vi "Instru.vi"(8 "错误输入（无错误）":errorcluster, 11 "VISA资源名称":refnum<visa-resource-name>="COM2") -> (0 "error out":errorcluster caption="错误输出")   [LabVIEW 2014]
uses:
  <vilib>/Instr/_visa.llb/VISA Configure Serial Port (Instr).vi
panel:
  out "温度":dbl
  out "电流通道":dbl
  out "电压通道":dbl
  out "实验类型":string
  out "示波器试验频率":dbl
  in  "实时数据停止":bool
  out "实时数据":dbl[](array[numeric])
  out "NegativeDutyCycle":dbl
  out "PositiveDutyCycle":dbl
  out "NegWidth":dbl
  out "PosWidth":dbl
  out "Falltime":dbl
  out "RiseTime":dbl
  out "ACRMS":dbl
  in  "x 2":bool
  out "FREQ":dbl
  out "MIN":dbl
  out "RMS":dbl
  out "AMP":dbl
  out "Max":dbl
  out "PK2PK":dbl
  out "PERIOD":dbl
  in  "一键查询":bool
  in  "停止 2":bool
  out "错误输出 2":errorcluster caption="错误输出"
  in  "停止":bool
  in  "自动采集":bool
  in  "查询":bool
  in  "选项卡控件":T1(tab)
  in  "保存数据与截图":bool
  out "二维图片":picture
  out "处理中":u8(slide) scale=0.0..100.0
  in  "选择通道":u16(ring) items=["电压通道", "电流通道"]
  out "表格控件":string[][](table)
  out "表格控件 2":string[][](table)
  out "表格控件 3":string[][](table)
  out "表格控件 11":string[][](table)
  out "表格控件 12":string[][](table)
  out "表格控件 13":string[][](table)
  out "表格控件 14":string[][](table)
  out "表格控件 15":string[][](table)
  out "表格控件 16":string[][](table)
  out "表格控件 17":string[][](table)
  in  "电流通道":enum32{"CH1", " 2"}(radio)
  in  "电压通道":T2(radio)
  in  "FTP":bool
  in  "复位":bool
  in  "查询仪表信息":bool
  out "仪表信息 2":string
  in  "地址":refnum<visa-resource-name>="DPO5054-C012667"
  # "示波器"
  # "查询各通道的参数值"
  # "结果显示"
  # "交流通道采集"
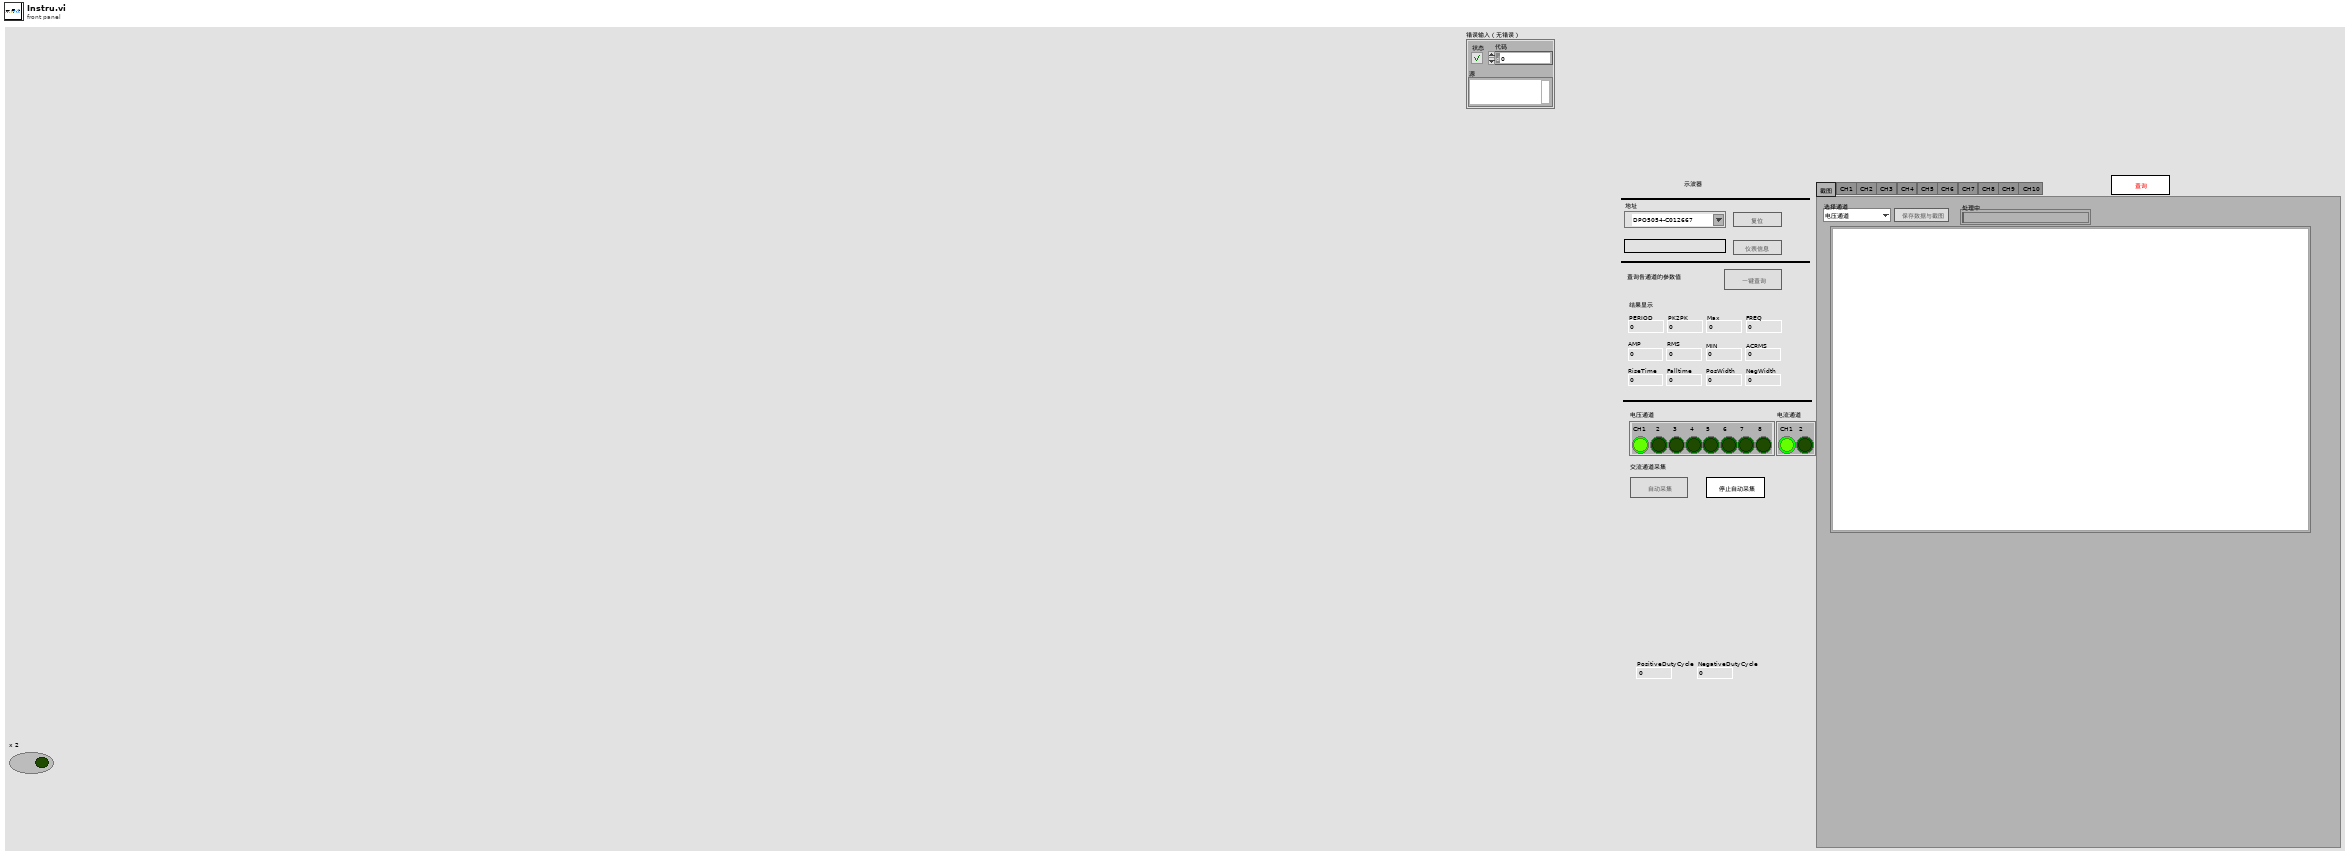
[diagram p1: front panel]
types:
  T1 = enum32{"截图", "CH1", "CH2", "CH3", "CH4", "CH5", "CH6", "CH7", "CH8", "CH9", "CH10"}
  T2 = enum32{"CH1", "2", "3", "4", " 5", " 6", " 7", " 8"}
  T3 = enum8{"Enabled", "Disabled", "Disabled and Grayed Out"}
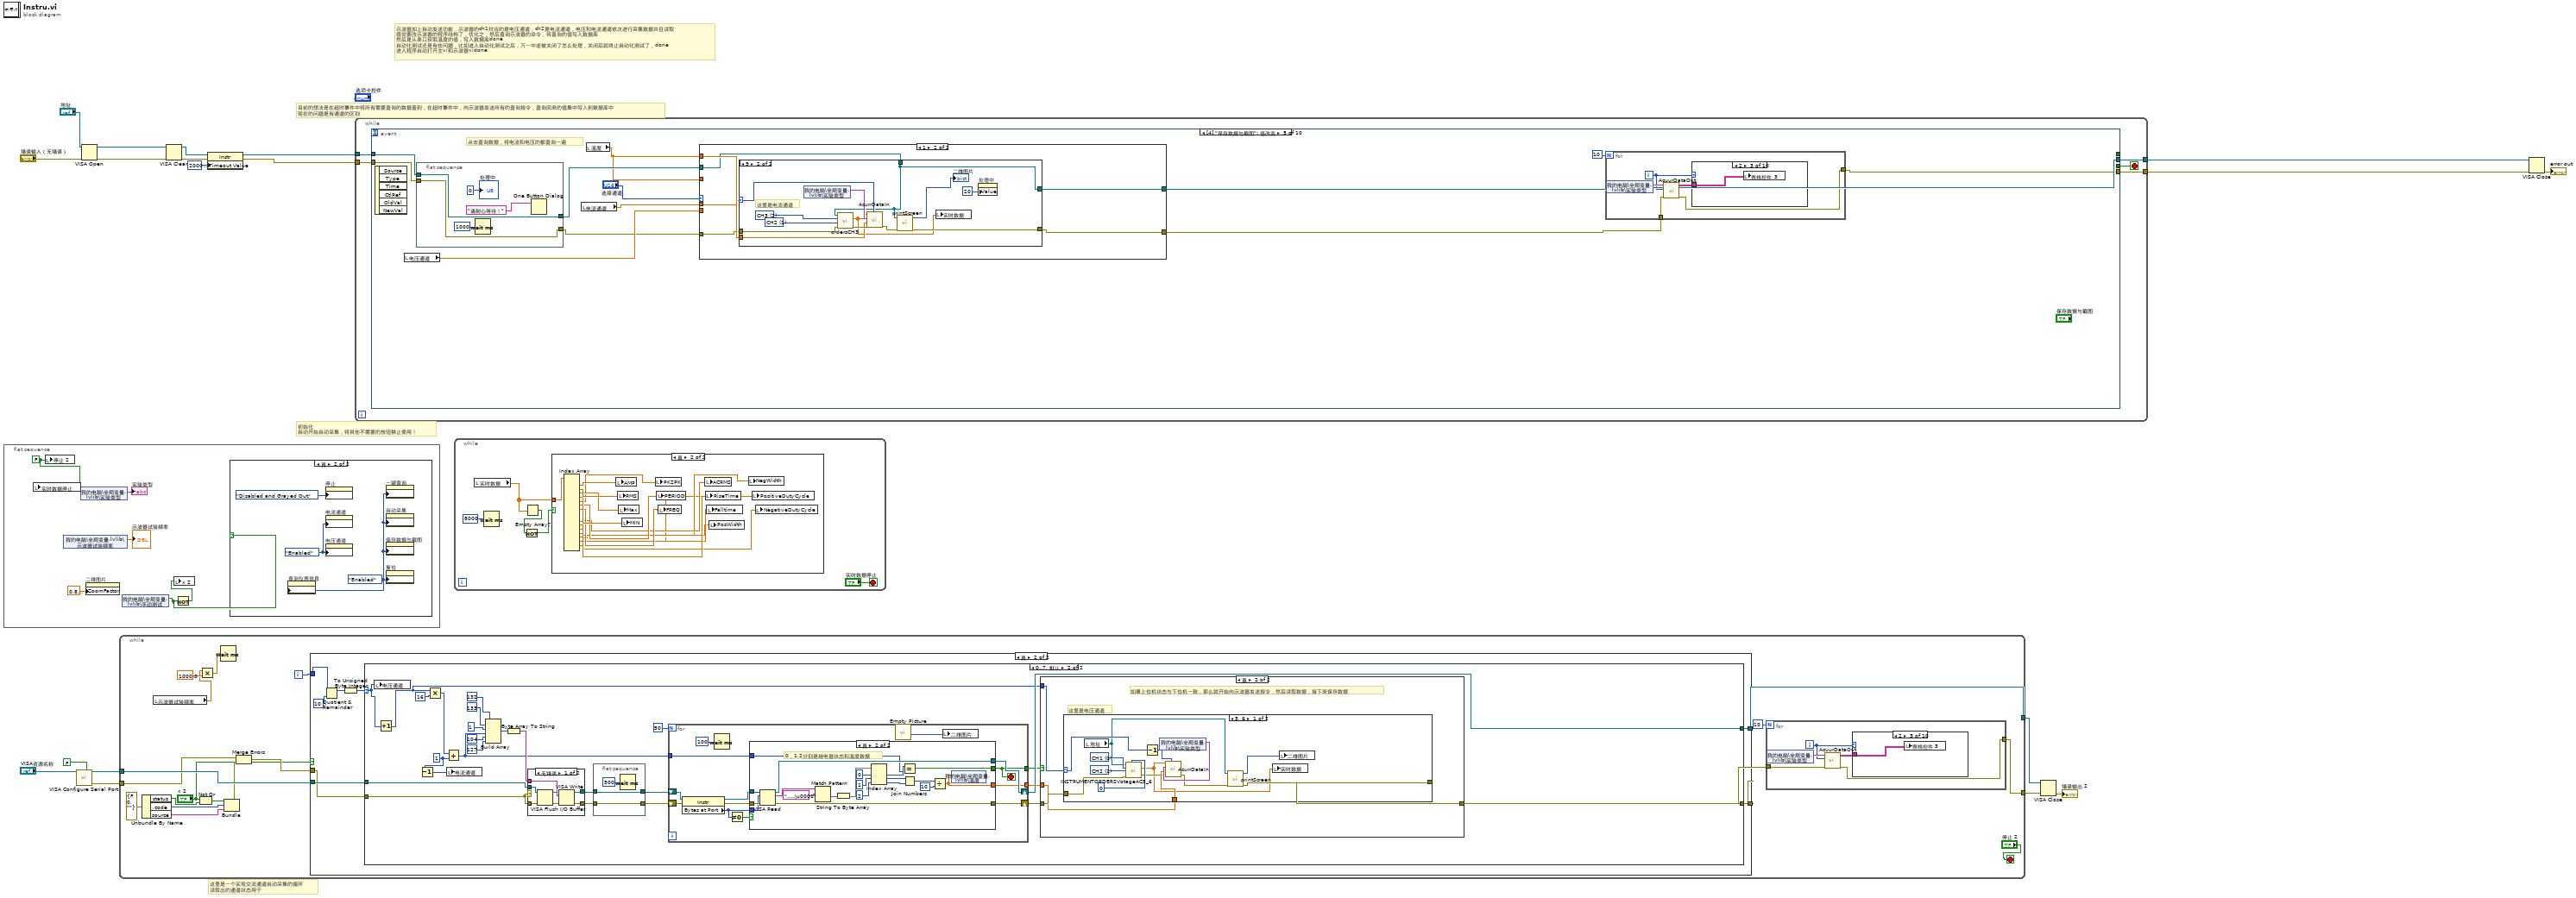
[diagram p0: block diagram]
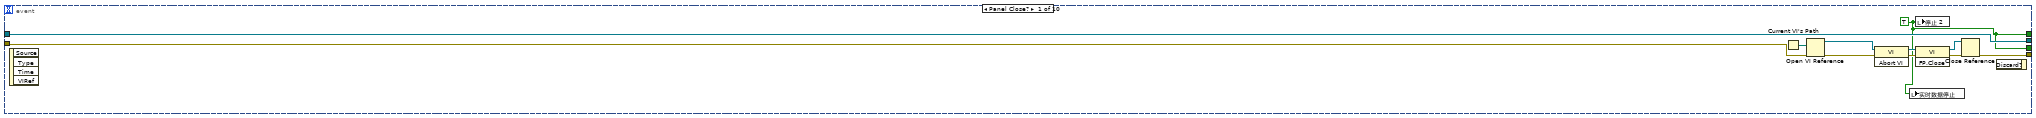
[diagram p3: hidden frame]
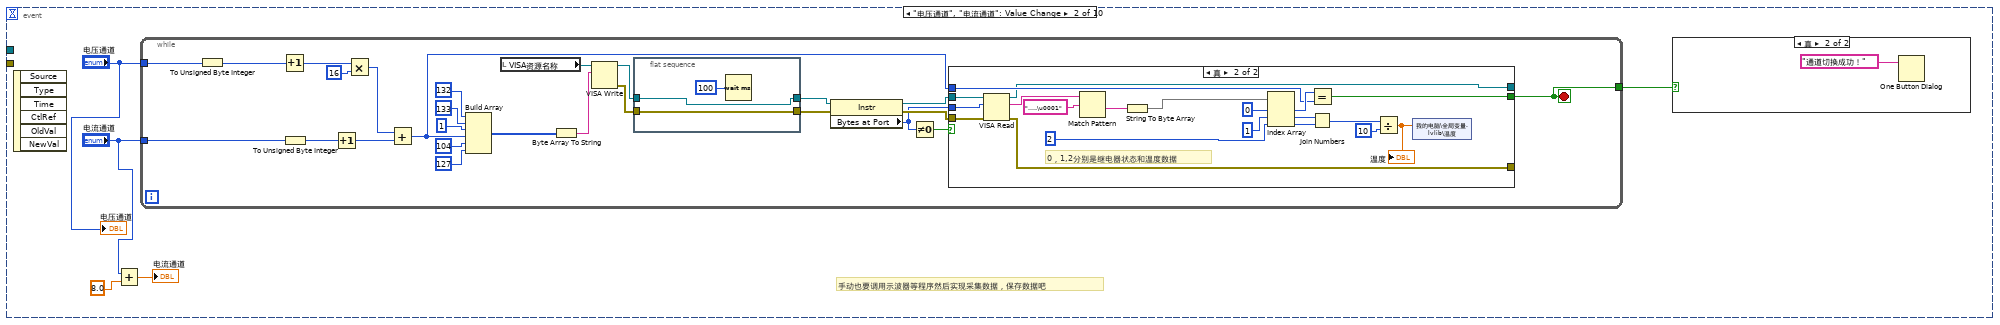
[diagram p4: hidden frame]
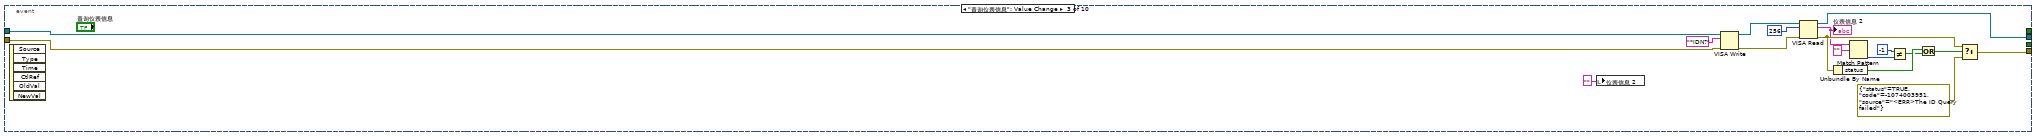
[diagram p7: hidden frame]
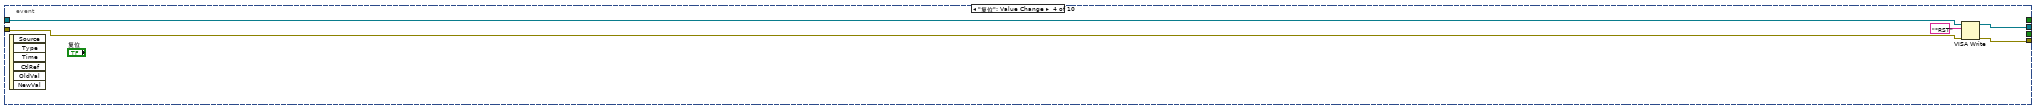
[diagram p8: hidden frame]
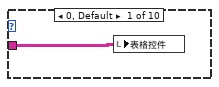
[diagram p9: hidden frame]
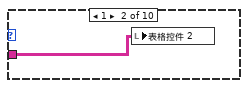
[diagram p10: hidden frame]
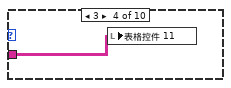
[diagram p11: hidden frame]
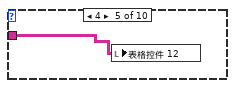
[diagram p12: hidden frame]
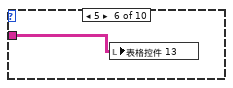
[diagram p13: hidden frame]
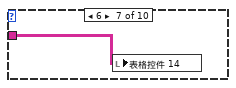
[diagram p14: hidden frame]
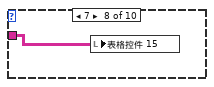
[diagram p15: hidden frame]
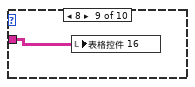
[diagram p16: hidden frame]
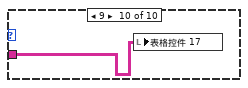
[diagram p17: hidden frame]
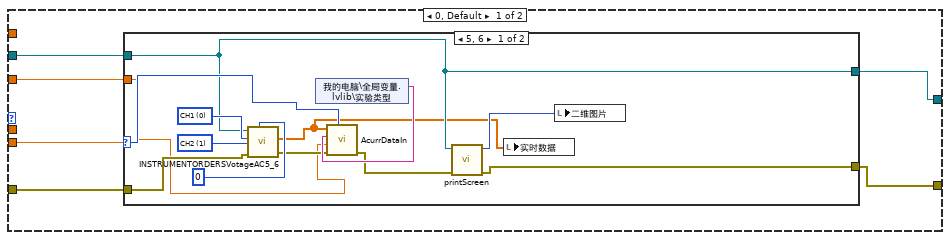
[diagram p18: hidden frame]
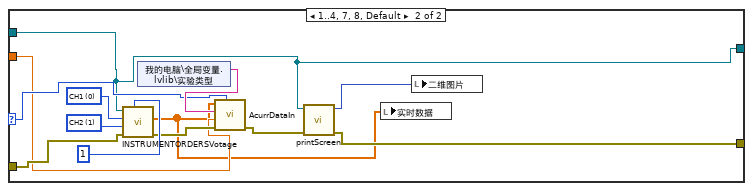
[diagram p19: hidden frame]
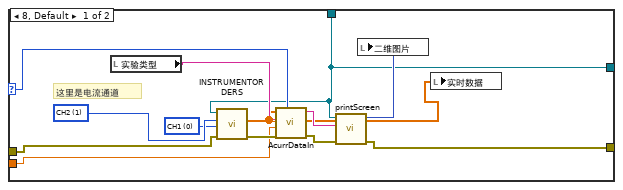
[diagram p20: hidden frame]
diagram:
  # "这里是一个实现交流通道自动采集的循环\n读取出的通道状态用于"
  # "目前的想法是在超时事件中将所有需要查询的数据查到，在超时事件中，向示波器发送所有的查询指令，查询回来的值集中写入到数据库中\n现在的问题是有通道的区别"
  # "初始化\n自动开始自动采集，将其他不需要的按钮禁止使用！"
  # "示波器加上自动发送功能，示波器的ch1对应的是电压通道，ch2是电流通道，电压和电流通道依次进行采集数据并且读取\n感觉要改示波器的程序结构了，优化之，然后查询示波器的命令，将查询的值写入数据库\n然后是从串口获取温度的值，写入数据库done\n自动化测试还是有些问题，比如进入自动化测试之后，万一中途被关闭了怎么处理，关闭后就终止自动化测试了，done\n进入程序自动打开主vi和示波器vidone"
  n1 = flat-sequence {
    frame #0 {
      w24 = FALSE
      n2 = local write "实时数据停止"(w24) -> ()
      n3 = local write "停止 2"(w24) -> ()
      n4 = shared-variable "我的电脑\\全局变量.lvlib\\示波器试验频率"() -> (→"示波器试验频率":dbl)  [unwired: 1 in, 1 out]
      n5 = shared-variable "我的电脑\\全局变量.lvlib\\实验类型"() -> (→"实验类型":string)  [unwired: 1 in, 1 out]
      n6 = property on="二维图片" class="Pict"("ZoomFactor"=sgl 0.8 ("缩放因子")) -> ()  [unwired: 2 in, 2 out]
      n7 = shared-variable "我的电脑\\全局变量.lvlib\\手动测试"() -> (w22:bool)  [unwired: 1 in, 1 out]
      n8 = Not(x=w22) -> (.not. x?=w23:bool)
      n9 = local write "x 2"(w23) -> ()
      n10 = case shown="真" w22 {
        frame False {
          w28 = T3."Disabled" ("禁用")
          w27 = T3."Disabled and Grayed Out" ("禁用")
          n11 = property on="停止" class="Bool"("DisabledEnum"=T3."Enabled" ("禁用")) -> ()  [unwired: 2 in, 2 out]
          n12 = property on="电流通道" class="RadioBtnsControl (严格)"("DisabledEnum"=w28) -> ()  [unwired: 2 in, 2 out]
          n13 = property on="电压通道" class="RadioBtnsControl (严格)"("DisabledEnum"=w28) -> ()  [unwired: 2 in, 2 out]
          n14 = property on="查询仪表信息" class="Bool"("DisabledEnum"=w27) -> ()  [unwired: 2 in, 2 out]
          n15 = property on="一键查询" class="Bool"("DisabledEnum"=w27) -> ()  [unwired: 2 in, 2 out]
          n16 = property on="自动采集" class="Bool"("DisabledEnum"=w27) -> ()  [unwired: 2 in, 2 out]
          n17 = property on="保存数据与截图" class="Bool"("DisabledEnum"=w27) -> ()  [unwired: 2 in, 2 out]
          n18 = property on="复位" class="Bool"("DisabledEnum"=w27) -> ()  [unwired: 2 in, 2 out]
        }
        frame True {
          w31 = T3."Enabled" ("禁用")
          w30 = T3."Enabled" ("禁用")
          n19 = property on="查询仪表信息" class="Bool"("DisabledEnum"=w30) -> ()  [unwired: 2 in, 2 out]
          n20 = property on="停止" class="Bool"("DisabledEnum"=T3."Disabled and Grayed Out" ("禁用")) -> ()  [unwired: 2 in, 2 out]
          n21 = property on="电流通道" class="RadioBtnsControl (严格)"("DisabledEnum"=w31) -> ()  [unwired: 2 in, 2 out]
          n22 = property on="电压通道" class="RadioBtnsControl (严格)"("DisabledEnum"=w31) -> ()  [unwired: 2 in, 2 out]
          n23 = property on="一键查询" class="Bool"("DisabledEnum"=w30) -> ()  [unwired: 2 in, 2 out]
          n24 = property on="自动采集" class="Bool"("DisabledEnum"=w30) -> ()  [unwired: 2 in, 2 out]
          n25 = property on="保存数据与截图" class="Bool"("DisabledEnum"=w30) -> ()  [unwired: 2 in, 2 out]
          n26 = property on="复位" class="Bool"("DisabledEnum"=w30) -> ()  [unwired: 2 in, 2 out]
        }
      }
    }
  }
  n27 = call-poly "VISA Configure Serial Port"("VISA resource name"="VISA资源名称", "Enable Termination\nChar (T)"=FALSE ("Enable Termination\nChar (T)")) -> ("VISA resource name out"=w15:refnum<visa-resource-name>, "error out"=w16:errorcluster)  [unwired: 12 in]
  n28 = VISA Open(error in (no error)="错误输入（无错误）", VISA resource name="地址") -> (VISA resource name=w8:refnum<visa-resource-name>, error out=w9:errorcluster)  [unwired: 3 in]
  n29 = while {
    tunnel: [w50] -> w1
    tunnel: w16 -> [w42]
    tunnel: w15 -> [w49]
    tunnel: [w35] -> w2
    i -> [w48]
    stop <- "停止 2" stop-if-true
    n30 = Unbundle By Name(errorcluster {"status"=FALSE, "code"=0, "source"=""} ("错误常量")) -> ("status"=w46:bool, "code"=w44:i32, "source"=w43:string)
    n31 = local read "示波器试验频率"() -> (w32:dbl)
    n32 = Not Or(1:w46, 2:"x 2") -> (0:w45:bool)
    n33 = Multiply(x=w32, y=1000.0) -> (x*y=w34:dbl)
    n34 = Wait (ms)(milliseconds to wait=w34) -> ()  [unwired: 1 out]
    n35 = Bundle(w45, "code"=w44, "source"=w43) -> (w41:cluster{bool, "code":i32, "source":string})  [unwired: 1 in]
    n36 = Merge Errors(w42, w41) -> (w40:errorcluster)
    n37 = case shown="真" "x 2" {
      tunnel: [_ w73] -> w50
      tunnel: w49 -> [_ w72]
      tunnel: [_ w66] -> w36
      tunnel: w48 -> [_ w69]
      tunnel: w40 -> [_ w67]
      frame False {
      }
      frame True {
        n38 = Quotient & Remainder(x=w69, y=10) -> (x-y*floor(x/y)=w70:i32)  [unwired: 1 out]
        n39 = To Unsigned Byte Integer(number=w70) -> (unsigned 8bit integer=w68:u8)
        n40 = case shown="0..7, 默认" w68 {
          selector: w68 -> [w82 w181]
          tunnel: [w80 w192] -> w73
          tunnel: w72 -> [w81 w191]
          tunnel: w67 -> [w79 w183]
          tunnel: [w74 w184] -> w66
          frame 8, 9 {
            w77 = u8 1
            # "然后将图片路径写入到数据库中即可，然后读需要的数据，然后直接写入到excel中就好了"
            # "如果上位机状态与下位机一致，那么就开始向示波器发送指令，然后读取数据，接下来保存数据"
            n41 = case shown="9, 默认" w82 {
              tunnel: [2 u8 1] -> w75
              frame 9, Default {
              }
              frame 8 {
              }
            }
            n42 = Decrement(x=w77) -> (x-1=w78:u8)
            n43 = local write "电压通道"(w78) -> ()
            n44 = Multiply(x=w77, y=u8 16) -> (x*y=w90:u8)
            n45 = Decrement(x=w75) -> (x-1=w76:i32)
            n46 = Add(x=w90, y=w75) -> (x+y=w88:i32)
            n47 = local write "电流通道"(w76) -> ()
            n48 = Build Array(u8 132, u8 133 ("元素"), u8 1 ("元素"), w88, u8 104 ("元素"), u8 127 ("元素")) -> (w96:i32[])
            n49 = Byte Array To String(unsigned byte array=w96) -> (string=w97:string)
            n50 = case shown="错误" w79 {
              tunnel: [w173 w175] -> w99
              tunnel: [w172 w174] -> w98
              tunnel: w97 -> [w171 _]
              tunnel: w79 -> [w170 w175]
              tunnel: w81 -> [w167 w174]
              frame No Error {
                n51 = VISA Flush I/O Buffer(VISA resource name=w167, error in (no error)=w170) -> (VISA resource name out=w169:refnum<visa-resource-name>, error out=w168:errorcluster)  [unwired: 1 in]
                n52 = VISA Write(VISA resource name=w169, write buffer=w171, error in (no error)=w168) -> (VISA resource name out=w172:refnum<visa-resource-name>, error out=w173:errorcluster)  [unwired: 1 out]
              }
              frame Error {
              }
            }
            n53 = flat-sequence {
              tunnel: w98 -> [w177]
              tunnel: [w177] -> w85
              tunnel: w99 -> [w176]
              tunnel: [w176] -> w100
              frame #0 {
                n54 = Wait (ms)(milliseconds to wait=u32 500 ("等待时间（毫秒）")) -> ()  [unwired: 1 out]
              }
            }
            n55 = for {
              N: 50 -> [_]
              tunnel: w88 -> [w108]
              tunnel: [w104] -> w87
              tunnel: [w107] -> w86
              shift-right: [w106] -> w83
              shift-left: w100 -> [w110]
              shift-right: [w109] -> w80
              shift-left: w85 -> [w105]
              stop <- w104 stop-if-true
              n56 = property class="Instr"(reference=w105, error in=w110) -> (reference out=w112:refnum<visa-resource-name>, error out=w113:errorcluster, "Bytes at Port"=w114:u32)
              n57 = Wait (ms)(milliseconds to wait=u32 100 ("等待时间（毫秒）")) -> ()  [unwired: 1 out]
              n58 = Not Equal To 0?(x=w114) -> (x != 0?=w111:bool)
              n59 = case shown="真" w111 {
                tunnel: w112 -> [w116 w136]
                tunnel: w113 -> [w115 w135]
                tunnel: w114 -> [_ w134]
                tunnel: [w116 w122] -> w109
                tunnel: [w115 w121] -> w106
                tunnel: w108 -> [_ w119]
                tunnel: [_ w118] -> w104
                tunnel: [_ w117] -> w107
                frame False {
                }
                frame True {
                  # "0，1,2分别是继电器状态和温度数据"
                  n60 = VISA Read(VISA resource name=w136, byte count=w134, error in (no error)=w135) -> (VISA resource name out=w122:refnum<visa-resource-name>, read buffer=w133:string, error out=w121:errorcluster)  [unwired: 1 out]
                  n61 = Match Pattern(string=w133, regular expression="…„\u0001" ("正则表达式")) -> (after substring=w131:string)  [unwired: 1 in, 3 out]
                  n62 = String To Byte Array(string=w131) -> (unsigned byte array=w130:u8[])
                  n63 = Index Array(array=w130, index #1=0 ("索引"), index #2=1 ("索引"), index #3=2 ("索引")) -> (element #1=w120:u8, element #2=w126:u8, element #3=w125:u8)
                  n64 = Equal?(x=w120, y=w119) -> (x = y?=w118:bool)
                  n65 = Join Numbers(hi=w126, lo=w125) -> ((hi.lo)=w124:u16)
                  n66 = Divide(x=w124, y=u16 10) -> (x/y=w117:dbl)
                  n67 = shared-variable "我的电脑\\全局变量.lvlib\\温度"(w117) -> ()  [unwired: 1 in, 1 out]
                }
              }
            }
            n68 = case shown="假" w87 {
              tunnel: w86 -> [_ w139]
              tunnel: w83 -> [w137 w140]
              tunnel: w82 -> [_ w138]
              tunnel: [w137 w141] -> w74
              frame False {
              }
              frame True {
                n69 = case shown="9" w138 {
                  selector: w138 -> [w144 w156]
                  tunnel: [w145 w166] -> w141
                  tunnel: w140 -> [w147 w162]
                  tunnel: w139 -> [w146 w159]
                  frame 8, Default {
                    w153 = u16 1 items=["CH1", "CH2", "CH3", "CH4"] ("通道选择 2")
                    w152 = u16 0 items=["CH1", "CH2", "CH3", "CH4"] ("通道选择 2")
                    # "这里是电流通道"
                    n70 = local read "实验类型"() -> (w142:string)
                    n71 = local read "地址"() -> (w154:refnum<visa-resource-name>)
                    n72 = call "INSTRUMENTORDERS.vi"("错误输入（无错误）"=w147, "关闭通道"=w152, "打开通道"=w153, "VISA资源名称"=w154) -> ("错误输出"=w150:errorcluster, "输出数组"=w151:dbl[])  [unwired: 5 in]
                    "实时数据" <- w151
                    n73 = call "AcurrDataIn.vi"("通道"=w144, "error in (no error)"=w150, "温度"=w146, "测试类型"=w142, "数组"=w151) -> ("error out"=w149:errorcluster, "记录时间"=w143:string)  [unwired: 5 in]
                    n74 = call "printScreen.vi"("错误输出"=w149, "记录时间"=w143, "地址"=w154) -> ("error out"=w145:errorcluster, "二维图片"=w148:picture)  [unwired: 6 in, 1 out]
                    n75 = local write "二维图片"(w148) -> ()
                  }
                  frame 9 {
                    w164 = u16 2 items=["CH1", "CH2", "CH3", "CH4"] ("通道选择 2")
                    w163 = u16 1 items=["CH1", "CH2", "CH3", "CH4"] ("通道选择 2")
                    # "这里是电流通道"
                    n76 = shared-variable "我的电脑\\全局变量.lvlib\\实验类型"() -> (w160:string)  [unwired: 1 in, 1 out]
                    n77 = local read "地址"() -> (w165:refnum<visa-resource-name>)
                    n78 = call "ordersCH3.vi"("错误输入（无错误）"=w162, "关闭通道"=w163, "打开通道"=w164, "VISA资源名称"=w165) -> ("错误输出"=w161:errorcluster, "输出数组"=w155:dbl[])  [unwired: 6 in]
                    n79 = call "AcurrDataIn.vi"("通道"=w156, "error in (no error)"=w161, "温度"=w159, "测试类型"=w160, "数组"=w155) -> ("error out"=w158:errorcluster)  [unwired: 5 in, 1 out]
                    n80 = call "printScreen.vi"("错误输出"=w158, "地址"=w165) -> ("error out"=w166:errorcluster, "二维图片"=w157:picture)  [unwired: 7 in, 1 out]
                    n81 = local write "二维图片"(w157) -> ()
                    n82 = local write "实时数据"(w155) -> ()
                  }
                }
              }
            }
          }
          frame 0..7, Default {
            w180 = u8 1
            n83 = local write "电压通道"(w181) -> ()
            n84 = Increment(x=w181) -> (x+1=w182:u8)
            n85 = Decrement(x=w180) -> (x-1=w179:u8)
            n86 = Multiply(x=w182, y=u8 16) -> (x*y=w194:u8)
            n87 = Add(x=w194, y=w180) -> (x+y=w190:u8)
            n88 = local write "电流通道"(w179) -> ()
            n89 = Build Array(u8 132, u8 133 ("元素"), u8 1 ("元素"), w190, u8 104 ("元素"), u8 127 ("元素")) -> (w200:u8[])
            n90 = Byte Array To String(unsigned byte array=w200) -> (string=w201:string)
            n91 = case shown="无错误" w183 {
              tunnel: [w278 w280] -> w203
              tunnel: [w277 w279] -> w202
              tunnel: w201 -> [w276 _]
              tunnel: w191 -> [w274 w279]
              tunnel: w183 -> [w275 w280]
              frame No Error {
                n92 = VISA Flush I/O Buffer(VISA resource name=w274, error in (no error)=w275) -> (VISA resource name out=w273:refnum<visa-resource-name>, error out=w272:errorcluster)  [unwired: 1 in]
                n93 = VISA Write(VISA resource name=w273, write buffer=w276, error in (no error)=w272) -> (VISA resource name out=w277:refnum<visa-resource-name>, error out=w278:errorcluster)  [unwired: 1 out]
              }
              frame Error {
              }
            }
            n94 = flat-sequence {
              tunnel: w202 -> [w282]
              tunnel: [w282] -> w187
              tunnel: w203 -> [w281]
              tunnel: [w281] -> w204
              frame #0 {
                n95 = Wait (ms)(milliseconds to wait=u32 500 ("等待时间（毫秒）")) -> ()  [unwired: 1 out]
              }
            }
            n96 = for {
              N: 50 -> [_]
              tunnel: w190 -> [w211]
              tunnel: [w207] -> w189
              tunnel: [w210] -> w188
              shift-right: [w209] -> w185
              shift-left: w204 -> [w213]
              shift-right: [w212] -> w192
              shift-left: w187 -> [w208]
              stop <- w207 stop-if-true
              n97 = property class="Instr"(reference=w208, error in=w213) -> (reference out=w215:refnum<visa-resource-name>, error out=w216:errorcluster, "Bytes at Port"=w217:u32)
              n98 = Wait (ms)(milliseconds to wait=u32 100 ("等待时间（毫秒）")) -> ()  [unwired: 1 out]
              n99 = Not Equal To 0?(x=w217) -> (x != 0?=w214:bool)
              n100 = case shown="真" w214 {
                tunnel: w215 -> [w219 w239]
                tunnel: w216 -> [w218 w238]
                tunnel: w217 -> [_ w237]
                tunnel: [w219 w225] -> w212
                tunnel: [w218 w224] -> w209
                tunnel: w211 -> [_ w222]
                tunnel: [_ w221] -> w207
                tunnel: [_ w220] -> w210
                frame False {
                }
                frame True {
                  # "0，1,2分别是继电器状态和温度数据"
                  n101 = VISA Read(VISA resource name=w239, byte count=w237, error in (no error)=w238) -> (VISA resource name out=w225:refnum<visa-resource-name>, read buffer=w236:string, error out=w224:errorcluster)  [unwired: 1 out]
                  n102 = Match Pattern(string=w236, regular expression="…„\u0001" ("正则表达式")) -> (after substring=w234:string)  [unwired: 1 in, 3 out]
                  n103 = String To Byte Array(string=w234) -> (unsigned byte array=w233:u8[])
                  n104 = Index Array(array=w233, index #1=0 ("索引"), index #2=1 ("索引"), index #3=2 ("索引")) -> (element #1=w223:u8, element #2=w229:u8, element #3=w228:u8)
                  n105 = Equal?(x=w223, y=w222) -> (x = y?=w221:bool)
                  n106 = Join Numbers(hi=w229, lo=w228) -> ((hi.lo)=w227:u16)
                  n107 = Divide(x=w227, y=u16 10) -> (x/y=w220:dbl)
                  n108 = shared-variable "我的电脑\\全局变量.lvlib\\温度"(w220) -> ()  [unwired: 1 in, 1 out]
                }
              }
              n109 = call "Empty Picture"() -> ("empty picture"=w205:picture)
              n110 = local write "二维图片"(w205) -> ()
            }
            n111 = case shown="真" w189 {
              tunnel: w188 -> [_ w241]
              tunnel: w185 -> [_ w242]
              tunnel: [_ w240] -> w184
              tunnel: w182 -> [_ w243]
              frame False {
              }
              frame True {
                # "这里是电压通道"
                # "如果上位机状态与下位机一致，那么就开始向示波器发送指令，然后读取数据，接下来保存数据"
                n112 = case shown="5, 6" w243 {
                  selector: w243 -> [w257 w271]
                  tunnel: w242 -> [w253 w266]
                  tunnel: w241 -> [w250 w263]
                  tunnel: [w256 w270] -> w240
                  frame 5, 6 {
                    w254 = u16 1 items=["CH1", "CH2", "CH3", "CH4"] ("通道选择 2")
                    w255 = u16 0 items=["CH1", "CH2", "CH3", "CH4"] ("通道选择 2")
                    n113 = local read "地址"() -> (w246:refnum<visa-resource-name>)
                    n114 = call "INSTRUMENTORDERSVotageAC5_6.vi"("行索引"=0, "错误输入（无错误）"=w253, "关闭通道"=w254, "打开通道"=w255, "VISA资源名称"=w246) -> ("错误输出"=w249:errorcluster, "输出数组"=w244:dbl[])  [unwired: 5 in]
                    n115 = Decrement(x=w257) -> (x-1=w248:u8)
                    n116 = shared-variable "我的电脑\\全局变量.lvlib\\实验类型"() -> (w251:string)  [unwired: 1 in, 1 out]
                    n117 = call "AcurrDataIn.vi"("通道"=w248, "error in (no error)"=w249, "温度"=w250, "测试类型"=w251, "数组"=w244) -> ("error out"=w247:errorcluster)  [unwired: 5 in, 1 out]
                    n118 = call "printScreen.vi"("错误输出"=w247, "地址"=w246) -> ("error out"=w256:errorcluster, "二维图片"=w245:picture)  [unwired: 7 in, 1 out]
                    n119 = local write "实时数据"(w244) -> ()
                    n120 = local write "二维图片"(w245) -> ()
                  }
                  frame 1..4, 7, 8, Default {
                    w268 = u16 1 items=["CH1", "CH2", "CH3", "CH4"] ("通道选择 2")
                    w269 = u16 0 items=["CH1", "CH2", "CH3", "CH4"] ("通道选择 2")
                    n121 = Decrement(x=w271) -> (x-1=w260:u8)
                    n122 = local read "地址"() -> (w261:refnum<visa-resource-name>)
                    n123 = call "INSTRUMENTORDERSVotage.vi"("行索引"=1, "错误输入（无错误）"=w266, "关闭通道"=w268, "打开通道"=w269, "VISA资源名称"=w261) -> ("错误输出"=w265:errorcluster, "输出数组"=w258:dbl[])  [unwired: 5 in]
                    n124 = shared-variable "我的电脑\\全局变量.lvlib\\实验类型"() -> (w264:string)  [unwired: 1 in, 1 out]
                    n125 = call "AcurrDataIn.vi"("通道"=w260, "error in (no error)"=w265, "温度"=w263, "测试类型"=w264, "数组"=w258) -> ("error out"=w262:errorcluster)  [unwired: 5 in, 1 out]
                    n126 = call "printScreen.vi"("错误输出"=w262, "地址"=w261) -> ("error out"=w270:errorcluster, "二维图片"=w259:picture)  [unwired: 7 in, 1 out]
                    n127 = local write "实时数据"(w258) -> ()
                    n128 = local write "二维图片"(w259) -> ()
                  }
                }
              }
            }
          }
        }
      }
    }
    n129 = for {
      N: 10 -> [_]
      tunnel: [w52] -> w35
      tunnel: w36 -> [w51]
      i -> [w54]
      n130 = shared-variable "我的电脑\\全局变量.lvlib\\实验类型"() -> (w55:string)  [unwired: 1 in, 1 out]
      n131 = call "AcuurDataOut.vi"("error in (no error)"=w51, "通道"=w54, "测试类型"=w55) -> ("error out 2"=w52:errorcluster, "表格控件 2"=w53:string[][])  [unwired: 7 in]
      n132 = case shown="2" w54 {
        tunnel: w53 -> [w56 w57 w58 w59 w60 w61 w62 w63 w64 w65]
        frame 0, Default {
          n133 = local write "表格控件"(w56) -> ()
        }
        frame 1 {
          n134 = local write "表格控件 2"(w57) -> ()
        }
        frame 2 {
          n135 = local write "表格控件 3"(w58) -> ()
        }
        frame 3 {
          n136 = local write "表格控件 11"(w59) -> ()
        }
        frame 4 {
          n137 = local write "表格控件 12"(w60) -> ()
        }
        frame 5 {
          n138 = local write "表格控件 13"(w61) -> ()
        }
        frame 6 {
          n139 = local write "表格控件 14"(w62) -> ()
        }
        frame 7 {
          n140 = local write "表格控件 15"(w63) -> ()
        }
        frame 8 {
          n141 = local write "表格控件 16"(w64) -> ()
        }
        frame 9 {
          n142 = local write "表格控件 17"(w65) -> ()
        }
      }
    }
  }
  n143 = VISA Clear(VISA resource name=w8, error in (no error)=w9) -> (VISA resource name out=w10:refnum<visa-resource-name>, error out=w11:errorcluster)
  n144 = property class="Instr"(reference=w10, error in=w11, "General Settings:Timeout Value"=u32 2000) -> (reference out=w5:refnum<visa-resource-name>, error out=w4:errorcluster)
  n145 = while {
    tunnel: w5 -> [w288]
    tunnel: [w286] -> w13
    tunnel: w4 -> [w287]
    tunnel: [w285] -> w14
    stop <- w284 stop-if-true
    n146 = event shown="[4] \"保存数据与截图\": 值改变" {
      selector: _ -> [_ _ _ _ _ _ _ _ _ _]
      dyn-events: _ -> [_ _ _ _ _ _ _ _ _ _]
      timeout: _ -> [_ _ _ _ _ _ _ _ _ _]
      tunnel: w288 -> [w299 _ w361 w378 w391 _ _ _ _ _]
      tunnel: w287 -> [w293 _ w360 w377 w390 w477 w479 _ _ _]
      tunnel: [w299 _ w359 w375 w383 _ _ _ _ _] -> w286
      tunnel: [w290 _ w358 w376 w380 w476 w478 _ _ _] -> w285
      tunnel: [w289 _ _ _ _ _ _ _ _ _] -> _
      tunnel: [w289 _ _ _ _ _ _ _ _ _] -> w284
      event Panel Close? {
        w289 = TRUE
        n147 = event-data() -> ()  [unwired: 1 in, 4 out]
        n148 = Current VI's Path() -> (path=w294:path)
        n149 = Open VI Reference(vi path=w294, error in (no error)=w293) -> (vi reference=w295:refnum<vi>, error out=w296:errorcluster)  [unwired: 4 in]
        n150 = invoke class="VI" method="Abort VI"(reference=w295, error in=w296) -> (reference out=w292:refnum<vi>, error out=w291:errorcluster)  [unwired: 1 in, 1 out]
        n151 = local write "实时数据停止"(w289) -> ()
        n152 = local write "停止 2"(w289) -> ()
        n153 = invoke class="VI" method="FP.Close"(reference=w292, error in=w291) -> (reference out=w298:refnum<vi>, error out=w297:errorcluster)  [unwired: 1 in, 1 out]
        n154 = Close Reference(reference=w298, error in (no error)=w297) -> (error out=w290:errorcluster)
        n155 = event-data() -> ()  [unwired: 2 in, 1 out]
      }
      event "电压通道", "电流通道": Value Change {
        # "手动也要调用示波器等程序然后实现采集数据，保存数据吧"
        n156 = event-data() -> ()  [unwired: 1 in, 6 out]
        n157 = Add(x="电流通道", y=8.0) -> (x+y=→"电流通道":dbl)
        n158 = while {
          tunnel: "电压通道" -> [w329]
          tunnel: "电流通道" -> [w328]
          tunnel: [w307] -> w304
          stop <- w307 stop-if-true
          n159 = To Unsigned Byte Integer(number=w329) -> (unsigned 8bit integer=w331:u8)
          n160 = Increment(x=w331) -> (x+1=w308:u8)
          n161 = To Unsigned Byte Integer(number=w328) -> (unsigned 8bit integer=w330:u8)
          n162 = Increment(x=w330) -> (x+1=w309:u8)
          n163 = Multiply(x=w308, y=u8 16) -> (x*y=w326:u8)
          n164 = Add(x=w326, y=w309) -> (x+y=w310:u8)
          n165 = Build Array(u8 132, u8 133 ("元素"), u8 1 ("元素"), w310, u8 104 ("元素"), u8 127 ("元素")) -> (w320:u8[])
          n166 = local read "VISA资源名称"() -> (w306:refnum<visa-resource-name>)
          n167 = Byte Array To String(unsigned byte array=w320) -> (string=w319:string)
          n168 = VISA Write(VISA resource name=w306, write buffer=w319) -> (VISA resource name out=w318:refnum<visa-resource-name>, error out=w317:errorcluster)  [unwired: 1 in, 1 out]
          n169 = flat-sequence {
            tunnel: w318 -> [w355]
            tunnel: [w355] -> w316
            tunnel: w317 -> [w354]
            tunnel: [w354] -> w315
            frame #0 {
              n170 = Wait (ms)(milliseconds to wait=u32 100 ("等待时间（毫秒）")) -> ()  [unwired: 1 out]
            }
          }
          n171 = property class="Instr"(reference=w316, error in=w315) -> (reference out=w313:refnum<visa-resource-name>, error out=w312:errorcluster, "Bytes at Port"=w311:u32)
          n172 = Not Equal To 0?(x=w311) -> (x != 0?=w314:bool)
          n173 = case shown="真" w314 {
            tunnel: w313 -> [w333 w353]
            tunnel: w312 -> [w332 w352]
            tunnel: w311 -> [_ w351]
            tunnel: w310 -> [_ w337]
            tunnel: [_ w336] -> w307
            tunnel: [w333 w335] -> _
            tunnel: [w332 w334] -> _
            frame False {
            }
            frame True {
              # "0，1,2分别是继电器状态和温度数据"
              n174 = VISA Read(VISA resource name=w353, byte count=w351, error in (no error)=w352) -> (VISA resource name out=w335:refnum<visa-resource-name>, read buffer=w350:string, error out=w334:errorcluster)  [unwired: 1 out]
              n175 = Match Pattern(string=w350, regular expression="…„\u0001" ("正则表达式")) -> (after substring=w348:string)  [unwired: 1 in, 3 out]
              n176 = String To Byte Array(string=w348) -> (unsigned byte array=w347:u8[])
              n177 = Index Array(array=w347, index #1=0 ("索引"), index #2=1 ("索引"), index #3=2 ("索引")) -> (element #1=w338:u8, element #2=w343:u8, element #3=w342:u8)
              n178 = Equal?(x=w338, y=w337) -> (x = y?=w336:bool)
              n179 = Join Numbers(hi=w343, lo=w342) -> ((hi.lo)=w341:u16)
              n180 = Divide(x=w341, y=u16 10) -> (x/y=w339:dbl)
              "温度" <- w339
              n181 = shared-variable "我的电脑\\全局变量.lvlib\\温度"(w339) -> ()  [unwired: 1 in, 1 out]
            }
          }
        }
        n182 = case shown="真" w304 {
          frame False {
          }
          frame True {
            n183 = One Button Dialog(message="通道切换成功！" ("消息")) -> ()  [unwired: 1 in, 1 out]
          }
        }
        "电压通道" <- "电压通道"
      }
      event "查询仪表信息": Value Change {
        n184 = event-data() -> ()  [unwired: 1 in, 6 out]
        n185 = local write "仪表信息 2"("" ("仪表信息 2")) -> ()
        n186 = VISA Write(VISA resource name=w361, write buffer="*IDN?" ("写入缓冲区"), error in (no error)=w360) -> (VISA resource name out=w365:refnum<visa-resource-name>, error out=w366:errorcluster)  [unwired: 1 out]
        n187 = VISA Read(VISA resource name=w365, byte count=u32 256 ("字节总数"), error in (no error)=w366) -> (VISA resource name out=w359:refnum<visa-resource-name>, read buffer=w363:string, error out=w374:errorcluster)  [unwired: 1 out]
        "仪表信息 2" <- w363
        n188 = Unbundle By Name(w374) -> ("status"=w372:bool)
        n189 = Match Pattern(string=w363, regular expression="" ("正则表达式")) -> (offset past match=w369:i32)  [unwired: 1 in, 3 out]
        n190 = Not Equal?(x=-1, y=w369) -> (x != y?=w371:bool)
        n191 = Or(x=w372, y=w371) -> (x .or. y?=w373:bool)
        n192 = Select(t=w374, s=w373, f=errorcluster {"status"=TRUE, "code"=-1074003951, "source"="<ERR>The ID Query failed"} ("错误常量")) -> (s? t:f=w358:errorcluster)
      }
      event "复位": Value Change {
        n193 = event-data() -> ()  [unwired: 1 in, 6 out]
        n194 = VISA Write(VISA resource name=w378, write buffer="*RST" ("写入缓冲区"), error in (no error)=w377) -> (VISA resource name out=w375:refnum<visa-resource-name>, error out=w376:errorcluster)  [unwired: 1 out]
      }
      event "保存数据与截图": Value Change {
        # "点击查询数据，将电流和电压的都查询一遍"
        n195 = event-data() -> ()  [unwired: 1 in, 6 out]
        n196 = local read "电压通道"() -> (w388:dbl)
        n197 = flat-sequence {
          tunnel: w391 -> [w474]
          tunnel: [w474] -> w387
          tunnel: w390 -> [w473]
          tunnel: [w473] -> w386
          frame #0 {
            n198 = Wait (ms)(milliseconds to wait=u32 1000 ("等待时间（毫秒）")) -> ()  [unwired: 1 out]
            n199 = One Button Dialog(message="请耐心等待！" ("消息")) -> ()  [unwired: 1 in, 1 out]
            "处理中" <- u8 0 ("处理中")
          }
        }
        n200 = local read "电流通道"() -> (w384:dbl)
        n201 = local read "温度"() -> (w385:dbl)
        n202 = case shown="1" "选择通道" {
          tunnel: w388 -> [w412 _]
          tunnel: w387 -> [w411 w441]
          tunnel: w386 -> [w410 w443]
          tunnel: w385 -> [w409 _]
          tunnel: w385 -> [_ w444]
          tunnel: w384 -> [_ w442]
          tunnel: [w407 w440] -> w381
          tunnel: [w408 w439] -> w383
          frame 0, Default {
            n203 = case shown="5, 6" w412 {
              selector: w412 -> [w416 w429]
              tunnel: w410 -> [w422 w434]
              tunnel: [w425 w438] -> w407
              tunnel: w411 -> [w414 w427]
              tunnel: w409 -> [w415 w428]
              tunnel: [w414 w427] -> w408
              frame 5, 6 {
                w423 = u16 1 items=["CH1", "CH2", "CH3", "CH4"] ("通道选择 2")
                w424 = u16 0 items=["CH1", "CH2", "CH3", "CH4"] ("通道选择 2")
                n204 = call "INSTRUMENTORDERSVotageAC5_6.vi"("行索引"=0, "错误输入（无错误）"=w422, "关闭通道"=w423, "打开通道"=w424, "VISA资源名称"=w414) -> ("错误输出"=w419:errorcluster, "输出数组"=w413:dbl[])  [unwired: 5 in]
                n205 = shared-variable "我的电脑\\全局变量.lvlib\\实验类型"() -> (w420:string)  [unwired: 1 in, 1 out]
                n206 = call "AcurrDataIn.vi"("通道"=w416, "error in (no error)"=w419, "温度"=w415, "测试类型"=w420, "数组"=w413) -> ("error out"=w418:errorcluster)  [unwired: 5 in, 1 out]
                n207 = call "printScreen.vi"("错误输出"=w418, "地址"=w414) -> ("error out"=w425:errorcluster, "二维图片"=w417:picture)  [unwired: 7 in, 1 out]
                n208 = local write "实时数据"(w413) -> ()
                n209 = local write "二维图片"(w417) -> ()
              }
              frame 1..4, 7, 8, Default {
                w436 = u16 1 items=["CH1", "CH2", "CH3", "CH4"] ("通道选择 2")
                w437 = u16 0 items=["CH1", "CH2", "CH3", "CH4"] ("通道选择 2")
                n210 = call "INSTRUMENTORDERSVotage.vi"("行索引"=1, "错误输入（无错误）"=w434, "关闭通道"=w436, "打开通道"=w437, "VISA资源名称"=w427) -> ("错误输出"=w433:errorcluster, "输出数组"=w426:dbl[])  [unwired: 5 in]
                n211 = shared-variable "我的电脑\\全局变量.lvlib\\实验类型"() -> (w432:string)  [unwired: 1 in, 1 out]
                n212 = call "AcurrDataIn.vi"("通道"=w429, "error in (no error)"=w433, "温度"=w428, "测试类型"=w432, "数组"=w426) -> ("error out"=w431:errorcluster)  [unwired: 5 in, 1 out]
                n213 = call "printScreen.vi"("错误输出"=w431, "地址"=w427) -> ("error out"=w438:errorcluster, "二维图片"=w430:picture)  [unwired: 7 in, 1 out]
                n214 = local write "实时数据"(w426) -> ()
                n215 = local write "二维图片"(w430) -> ()
              }
            }
          }
          frame 1 {
            n216 = case shown="9" w442 {
              selector: w442 -> [w449 w462]
              tunnel: [w450 w470] -> w440
              tunnel: w443 -> [w452 w467]
              tunnel: w444 -> [w451 w464]
              tunnel: w441 -> [w446 w459]
              tunnel: [w446 w459] -> w439
              frame 8, Default {
                w457 = u16 1 items=["CH1", "CH2", "CH3", "CH4"] ("通道选择 2")
                w456 = u16 0 items=["CH1", "CH2", "CH3", "CH4"] ("通道选择 2")
                # "这里是电流通道"
                n217 = local read "实验类型"() -> (w447:string)
                n218 = call "INSTRUMENTORDERS.vi"("错误输入（无错误）"=w452, "关闭通道"=w456, "打开通道"=w457, "VISA资源名称"=w446) -> ("错误输出"=w455:errorcluster, "输出数组"=w445:dbl[])  [unwired: 5 in]
                n219 = call "AcurrDataIn.vi"("通道"=w449, "error in (no error)"=w455, "温度"=w451, "测试类型"=w447, "数组"=w445) -> ("error out"=w454:errorcluster, "记录时间"=w448:string)  [unwired: 5 in]
                n220 = call "printScreen.vi"("错误输出"=w454, "记录时间"=w448, "地址"=w446) -> ("error out"=w450:errorcluster, "二维图片"=w453:picture)  [unwired: 6 in, 1 out]
                n221 = local write "二维图片"(w453) -> ()
                n222 = local write "实时数据"(w445) -> ()
              }
              frame 9 {
                w469 = u16 2 items=["CH1", "CH2", "CH3", "CH4"] ("通道选择 2")
                w468 = u16 1 items=["CH1", "CH2", "CH3", "CH4"] ("通道选择 2")
                # "这里是电流通道"
                n223 = shared-variable "我的电脑\\全局变量.lvlib\\实验类型"() -> (w465:string)  [unwired: 1 in, 1 out]
                n224 = call "ordersCH3.vi"("错误输入（无错误）"=w467, "关闭通道"=w468, "打开通道"=w469, "VISA资源名称"=w459) -> ("错误输出"=w466:errorcluster, "输出数组"=w458:dbl[])  [unwired: 6 in]
                n225 = call "AcurrDataIn.vi"("通道"=w462, "error in (no error)"=w466, "温度"=w464, "测试类型"=w465, "数组"=w458) -> ("error out"=w463:errorcluster)  [unwired: 5 in, 1 out]
                n226 = call "printScreen.vi"("错误输出"=w463, "地址"=w459) -> ("error out"=w470:errorcluster, "二维图片"=→"二维图片":picture)  [unwired: 7 in, 1 out]
                n227 = local write "实时数据"(w458) -> ()
                n228 = property on="处理中" class="Slide (严格)"("Value"=u8 20 ("处理中")) -> ()  [unwired: 2 in, 2 out]
              }
            }
          }
        }
        n229 = for {
          N: 10 -> [_]
          tunnel: [w393] -> w380
          tunnel: w381 -> [w392]
          i -> [w395]
          n230 = shared-variable "我的电脑\\全局变量.lvlib\\实验类型"() -> (w396:string)  [unwired: 1 in, 1 out]
          n231 = call "AcuurDataOut.vi"("error in (no error)"=w392, "通道"=w395, "测试类型"=w396) -> ("error out 2"=w393:errorcluster, "表格控件 2"=w394:string[][])  [unwired: 7 in]
          n232 = case shown="2" w395 {
            tunnel: w394 -> [w397 w398 w399 w400 w401 w402 w403 w404 w405 w406]
            frame 0, Default {
              n233 = local write "表格控件"(w397) -> ()
            }
            frame 1 {
              n234 = local write "表格控件 2"(w398) -> ()
            }
            frame 2 {
              n235 = local write "表格控件 3"(w399) -> ()
            }
            frame 3 {
              n236 = local write "表格控件 11"(w400) -> ()
            }
            frame 4 {
              n237 = local write "表格控件 12"(w401) -> ()
            }
            frame 5 {
              n238 = local write "表格控件 13"(w402) -> ()
            }
            frame 6 {
              n239 = local write "表格控件 14"(w403) -> ()
            }
            frame 7 {
              n240 = local write "表格控件 15"(w404) -> ()
            }
            frame 8 {
              n241 = local write "表格控件 16"(w405) -> ()
            }
            frame 9 {
              n242 = local write "表格控件 17"(w406) -> ()
            }
          }
        }
      }
      event "FTP": Value Change {
        n243 = event-data() -> ()  [unwired: 1 in, 6 out]
        n244 = call "FTPTools.vi"("error in (no error)"=w477) -> ("error out"=w476:errorcluster)  [unwired: 10 in]
      }
      event "查询": Value Change {
        n245 = event-data() -> ()  [unwired: 1 in, 6 out]
        n246 = for {
          N: 10 -> [_]
          tunnel: w479 -> [w482]
          tunnel: [w481] -> w478
          i -> [w484]
          n247 = shared-variable "我的电脑\\全局变量.lvlib\\实验类型"() -> (w485:string)  [unwired: 1 in, 1 out]
          n248 = call "AcuurDataOut.vi"("error in (no error)"=w482, "通道"=w484, "测试类型"=w485) -> ("error out 2"=w481:errorcluster, "表格控件 2"=w483:string[][])  [unwired: 7 in]
          n249 = case shown="0, 默认" w484 {
            tunnel: w483 -> [w486 w487 w488 w489 w490 w491 w492 w493 w494 w495]
            frame 0, Default {
              "表格控件" <- w486
            }
            frame 1 {
              "表格控件 2" <- w487
            }
            frame 2 {
              "表格控件 3" <- w488
            }
            frame 3 {
              "表格控件 11" <- w489
            }
            frame 4 {
              "表格控件 12" <- w490
            }
            frame 5 {
              "表格控件 13" <- w491
            }
            frame 6 {
              "表格控件 14" <- w492
            }
            frame 7 {
              "表格控件 15" <- w493
            }
            frame 8 {
              "表格控件 16" <- w494
            }
            frame 9 {
              "表格控件 17" <- w495
            }
          }
        }
      }
      event "自动采集": Value Change {
        w497 = T3."Disabled" ("禁用")
        w498 = T3."Disabled and Grayed Out" ("禁用")
        n250 = event-data() -> ()  [unwired: 1 in, 6 out]
        n251 = local write "x 2"(TRUE) -> ()
        n252 = property on="停止" class="Bool"("DisabledEnum"=T3."Enabled" ("禁用")) -> ()  [unwired: 2 in, 2 out]
        n253 = property on="电流通道" class="RadioBtnsControl (严格)"("DisabledEnum"=w497) -> ()  [unwired: 2 in, 2 out]
        n254 = property on="电压通道" class="RadioBtnsControl (严格)"("DisabledEnum"=w497) -> ()  [unwired: 2 in, 2 out]
        n255 = property on="一键查询" class="Bool"("DisabledEnum"=w498) -> ()  [unwired: 2 in, 2 out]
        n256 = property on="自动采集" class="Bool"("DisabledEnum"=w498) -> ()  [unwired: 2 in, 2 out]
        n257 = property on="保存数据与截图" class="Bool"("DisabledEnum"=w498) -> ()  [unwired: 2 in, 2 out]
        n258 = property on="复位" class="Bool"("DisabledEnum"=w498) -> ()  [unwired: 2 in, 2 out]
        n259 = property on="查询仪表信息" class="Bool"("DisabledEnum"=w498) -> ()  [unwired: 2 in, 2 out]
      }
      event "停止": Value Change {
        n260 = event-data() -> ()  [unwired: 1 in, 6 out]
        n261 = flat-sequence {
          tunnel: [w504] -> w501
          tunnel: [w503] -> w500
          tunnel: w501 -> [w510]
          tunnel: w500 -> [w509]
          frame #0 {
            n262 = local write "x 2"(FALSE) -> ()
          }
          frame #1 {
            n263 = Current VI's Path() -> (path=w506:path)
            n264 = Wait (ms)(milliseconds to wait=u32 5000 ("等待时间（毫秒）")) -> ()  [unwired: 1 out]
            n265 = Open VI Reference(vi path=w506) -> (vi reference=w503:refnum<vi>)  [unwired: 5 in, 1 out]
            n266 = call <vilib>:"Set Busy.vi"("disable click? (T)"=TRUE, "VI reference (current VI)"=w503) -> ("error out"=w504:errorcluster)  [unwired: 8 in, 1 out]
          }
          frame #2 {
            w508 = T3."Enabled" ("禁用")
            w511 = T3."Enabled" ("禁用")
            n267 = call <vilib>:"Unset Busy.vi"("error in (no error)"=w510, "VI reference (current VI)"=w509) -> ()  [unwired: 9 in, 1 out]
            n268 = property on="电流通道" class="RadioBtnsControl (严格)"("DisabledEnum"=w508) -> ()  [unwired: 2 in, 2 out]
            n269 = property on="电压通道" class="RadioBtnsControl (严格)"("DisabledEnum"=w508) -> ()  [unwired: 2 in, 2 out]
            n270 = property on="一键查询" class="Bool"("DisabledEnum"=w511) -> ()  [unwired: 2 in, 2 out]
            n271 = property on="自动采集" class="Bool"("DisabledEnum"=w511) -> ()  [unwired: 2 in, 2 out]
            n272 = property on="保存数据与截图" class="Bool"("DisabledEnum"=w511) -> ()  [unwired: 2 in, 2 out]
            n273 = property on="复位" class="Bool"("DisabledEnum"=w511) -> ()  [unwired: 2 in, 2 out]
            n274 = property on="查询仪表信息" class="Bool"("DisabledEnum"=w511) -> ()  [unwired: 2 in, 2 out]
            n275 = One Button Dialog(message="已停止自动采集！") -> ()  [unwired: 1 in, 1 out]
            n276 = property on="停止" class="Bool"("DisabledEnum"=T3."Disabled and Grayed Out" ("禁用")) -> ()  [unwired: 2 in, 2 out]
          }
        }
      }
      event "一键查询": Value Change {
        n277 = event-data() -> ()  [unwired: 1 in, 6 out]
        n278 = local read "实时数据"() -> (w528:dbl[])
        n279 = Index Array(array=w528) -> (element #1=w527:dbl, element #2=w526:dbl, element #3=w525:dbl, element #4=w524:dbl, element #5=w523:dbl, element #6=w522:dbl, element #7=w521:dbl, element #10=w520:dbl, element #11=w519:dbl, element #12=w518:dbl, element #13=w517:dbl, element #14=w516:dbl, element #15=w515:dbl, element #16=w514:dbl)  [unwired: 17 in, 3 out]
        n280 = local write "AMP"(w527) -> ()
        n281 = local write "RMS"(w526) -> ()
        n282 = local write "Max"(w525) -> ()
        n283 = local write "MIN"(w524) -> ()
        n284 = local write "PK2PK"(w523) -> ()
        n285 = local write "PERIOD"(w522) -> ()
        n286 = local write "FREQ"(w521) -> ()
        n287 = local write "ACRMS"(w520) -> ()
        n288 = local write "RiseTime"(w519) -> ()
        n289 = local write "Falltime"(w518) -> ()
        n290 = local write "PosWidth"(w517) -> ()
        n291 = local write "NegWidth"(w516) -> ()
        n292 = local write "PositiveDutyCycle"(w515) -> ()
        n293 = local write "NegativeDutyCycle"(w514) -> ()
      }
    }
  }
  n294 = while {
    stop <- "实时数据停止" stop-if-true
    n295 = local read "实时数据"() -> (w529:dbl[])
    n296 = Wait (ms)(milliseconds to wait=u32 8000 ("等待时间（毫秒）")) -> ()  [unwired: 1 out]
    n297 = Empty Array?(array=w529) -> (empty?=w531:bool)
    n298 = Not(x=w531) -> (.not. x?=w530:bool)
    n299 = case shown="真" w530 {
      tunnel: w529 -> [_ w534]
      frame False {
      }
      frame True {
        n300 = Index Array(array=w534) -> (element #1=w548:dbl, element #2=w547:dbl, element #3=w546:dbl, element #4=w545:dbl, element #5=w544:dbl, element #6=w543:dbl, element #7=w542:dbl, element #10=w541:dbl, element #11=w540:dbl, element #12=w539:dbl, element #13=w538:dbl, element #14=w537:dbl, element #15=w536:dbl, element #16=w535:dbl)  [unwired: 17 in, 3 out]
        n301 = local write "AMP"(w548) -> ()
        n302 = local write "RMS"(w547) -> ()
        n303 = local write "Max"(w546) -> ()
        n304 = local write "MIN"(w545) -> ()
        n305 = local write "PK2PK"(w544) -> ()
        n306 = local write "PERIOD"(w543) -> ()
        n307 = local write "FREQ"(w542) -> ()
        n308 = local write "ACRMS"(w541) -> ()
        n309 = local write "RiseTime"(w540) -> ()
        n310 = local write "Falltime"(w539) -> ()
        n311 = local write "PosWidth"(w538) -> ()
        n312 = local write "NegWidth"(w537) -> ()
        n313 = local write "PositiveDutyCycle"(w536) -> ()
        n314 = local write "NegativeDutyCycle"(w535) -> ()
      }
    }
  }
  n315 = VISA Close(VISA resource name=w1, error in (no error)=w2) -> (error out=→"错误输出 2":errorcluster)
  n316 = VISA Close(VISA resource name=w13, error in (no error)=w14) -> (error out=→"error out":errorcluster)
